vi "StartTestSuite_AfterEndTestSuite_AddsSiblingTestSuite.vi"() -> (0 "error out":errorcluster)   [LabVIEW 2017, in "ResultTreeListener.Tests.lvlib"]
uses:
  ResultTreeListener.Tests.lvlib
  6b75ad31-72ea-41ab-b928-28c96779d91c.vi
  Support/FakeTestSuite/FakeTestSuite.lvclass
  C:/Users/de200256/Code/logmanoriginal/lvunit/TestSuite/TestSuite.lvclass
  Constraint/IsEqual/Create.vi
  ResultTreeListener/ResultTreeListener.lvclass
  Constraint/IsEqual/IsEqual.lvclass
  ResultTree/ResultTree.lvclass
panel:
  in  "Tree":string(tree)
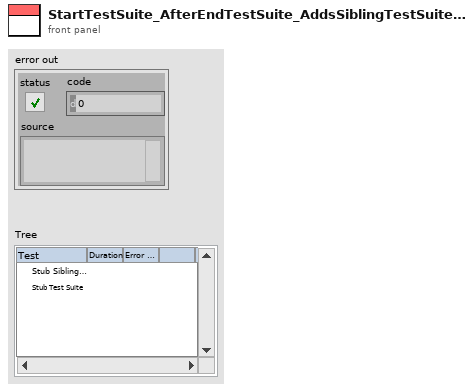
[diagram p1: front panel]
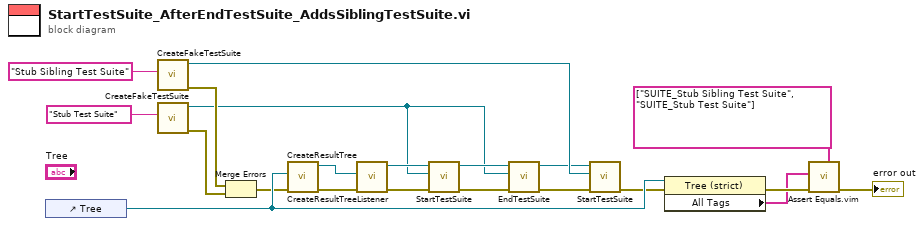
[diagram p0: block diagram]
diagram:
  n1 = control-ref of="Tree"() -> (w14:refnum<vi>)
  n2 = call "CreateFakeTestSuite.vi"("Name"="Stub Sibling Test Suite") -> ("error out"=w6:errorcluster, "FakeTestSuite out"=w8:refnum<class "FakeTestSuite.lvclass">)  [unwired: 9 in]
  n3 = call "CreateFakeTestSuite.vi"("Name"="Stub Test Suite") -> ("error out"=w5:errorcluster, "FakeTestSuite out"=w1:refnum<class "FakeTestSuite.lvclass">)  [unwired: 9 in]
  n4 = Merge Errors(w6, w5) -> (w7:errorcluster)
  n5 = call "CreateResultTree.vi"("error in (no error)"=w7, "Tree Refnum"=w14) -> ("error out"=w21:errorcluster, "ResultTree out"=w20:refnum<class "ResultTree.lvclass">)  [unwired: 8 in]
  n6 = call "CreateResultTreeListener.vi"("error in (no error)"=w21, "ResultTree"=w20) -> ("error out"=w19:errorcluster, "ResultTreeListener out"=w17:refnum<class "ResultTreeListener.lvclass">)  [unwired: 8 in]
  n7 = call-dynamic "StartTestSuite.vi"("error in (no error)"=w19, "TestSuite"=w1, "ResultTreeListener in"=w17) -> ("error out"=w10:errorcluster, "ResultTreeListener out"=w3:refnum<class "ResultTreeListener.lvclass">)  [unwired: 7 in]
  n8 = call-dynamic "EndTestSuite.vi"("error in (no error)"=w10, "TestSuite"=w1, "ResultTreeListener in"=w3) -> ("error out"=w4:errorcluster, "ResultTreeListener out"=w2:refnum<class "ResultTreeListener.lvclass">)  [unwired: 7 in]
  n9 = call-dynamic "StartTestSuite.vi"("error in (no error)"=w4, "TestSuite"=w8, "ResultTreeListener in"=w2) -> ("error out"=w9:errorcluster)  [unwired: 7 in, 1 out]
  n10 = property class="Tree (strict)"(reference=w14, error in=w9) -> (error out=w15:errorcluster, "All Tags"=w13:string[])  [unwired: 1 out]
  n11 = call "Assert Equals.vim"("Expected"=string[] ["SUITE_Stub Sibling Test Suite", "SUITE_Stub Test Suite"] ("All Tags"), "error in (no error)"=w15, "Actual"=w13) -> ("error out"=→"error out":errorcluster)  [unwired: 8 in]
